vi "pupil find 12 sub vi.vi"(4 "Curve Parameters":T3={"Extraction Mode"=0, "Edge Threshold"=1, "Edge Filter Size"=0, "Min Length"=25, "Row Search Step Size"=10, "Col Search Step Size"=10, "Max Endpoint Gap"=10, "Closed"=FALSE, "Subpixel"=TRUE} {"Max Endpoint Gap" min=0; "Col Search Step Size" min=1 max=255 step=1; "Row Search Step Size" min=1 max=255 step=1; "Min Length" min=0; "Edge Filter Size" items=["Fine", "Normal", "Controur Tracing"]; "Edge Threshold" min=1 max=65535 step=1; "Extraction Mode" items=["Normal", "Uniform Regions"]}, 6 "Circle Descriptor":cluster{"Min Radius":dbl, "Max Radius":dbl}, 7 "New Image 2":T2, 9 "threshold":cluster{"Lower value":sgl, "Upper value":sgl}, 10 "New Image":T2, 11 "Refnum in":T2) -> (0 "Circles":T1(array[cluster]) {"Position"."Y" format="%.2f"; "Position"."X" format="%.2f"}, 1 "Radius":dbl, 2 "Image Dst Out":T2, 3 "Refnum out":T2)   [LabVIEW 2023]
uses:
  <vilib>/vision/Pattern Matching.llb/IMAQ Curve Parameters.ctl
  <vilib>/vision/Image Controls.llb/IMAQ Image.ctl
  <vilib>/vision/Shape Detection.llb/ShapeDetectionMatchOptions.ctl
  <vilib>/vision/Pattern Matching.llb/IMAQ Match Range Setting.ctl
  <vilib>/vision/NI_Vision_Development_Module.lvlib
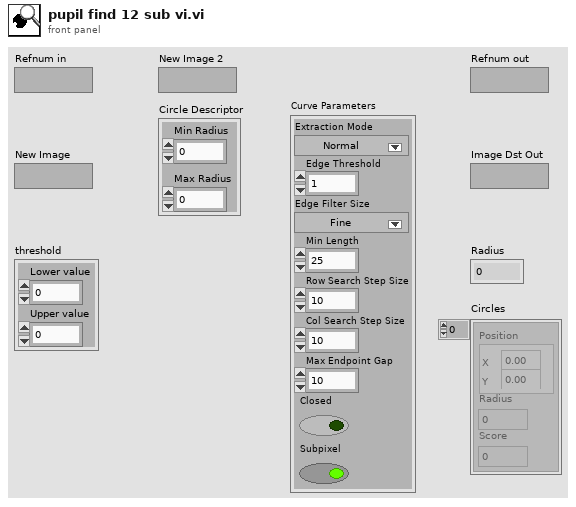
[diagram p1: front panel]
types:
  T1 = cluster{"Position":cluster{"X":sgl, "Y":sgl}, "Radius":dbl, "Score":dbl}[]
  T2 = typedef "IMAQ Image.ctl" = refnum<image>
  T3 = typedef "IMAQ Curve Parameters.ctl" = cluster{"Extraction Mode":u32, "Edge Threshold":i32, "Edge Filter Size":u32, "Min Length":i32, "Row Search Step Size":i32, "Col Search Step Size":i32, "Max Endpoint Gap":i32, "Closed":bool, "Subpixel":bool}
  T4 = typedef "ShapeDetectionMatchOptions.ctl" = cluster{"Rotation":bool, "Scale":bool, "Occlusion":bool, "Range Settings":T5[]}
  T5 = typedef "IMAQ Match Range Setting.ctl" = cluster{"Match Constraints":u32, "Min":dbl, "Max":dbl}
  T6 = typedef "IMAQ Circle" = cluster{"Center X":i32, "Center Y":i32, "Inner Radius":i32, "Outer Radius":i32, "Start Angle":dbl, "End Angle":dbl}
  T7 = typedef "ROI Descriptor" = cluster{"Global Rectangle":i32[], "Contours":cluster{"ID":enum32{"External", "Internal"}, "Type":u32, "Coordinates":i32[]}[]}
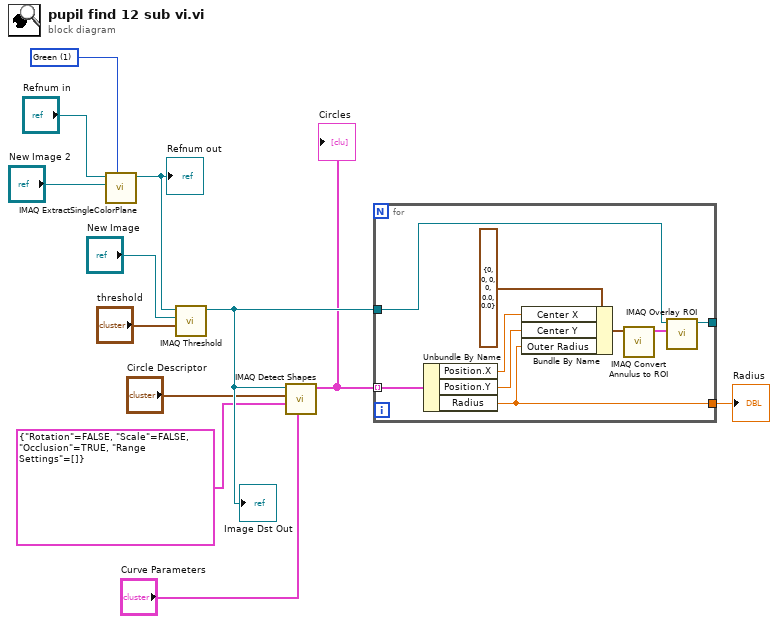
[diagram p0: block diagram]
diagram:
  w1 = 1 items=["Red", "Green", "Blue", "Hue", "Saturation", "Luminance", "Value", "Intensity"] ("Color Plane")
  n1 = call "IMAQ ExtractSingleColorPlane"("Color Plane"=w1, "Image Dst"="New Image 2", "Image Src"="Refnum in") -> ("Image Dst Out"=w6:T2)  [unwired: 7 in, 1 out]
  "Refnum out" <- w6
  n2 = call "IMAQ Threshold"("Range"="threshold", "Image Dst"="New Image", "Image Src"=w6) -> ("Image Dst Out"=w12:T2)  [unwired: 7 in, 1 out]
  "Image Dst Out" <- w12
  n3 = call-poly "IMAQ Detect Shapes"("Curve Parameters"="Curve Parameters", "Match Options"=T4 {"Rotation"=FALSE, "Scale"=FALSE, "Occlusion"=TRUE, "Range Settings"=[]}, "Circle Descriptor"="Circle Descriptor", "Image"=w12) -> ("Circles"=w7:T1)  [unwired: 5 in, 2 out]
  "Circles" <- w7
  n4 = for {
    tunnel: w12 -> [w16]
    tunnel: w7 -> [w15] mode=indexing
    tunnel: [w14] -> _
    tunnel: [w13] -> w11
    n5 = Unbundle By Name(w15) -> ("Position.X"=w19:sgl, "Position.Y"=w18:sgl, "Radius"=w13:dbl)
    n6 = Bundle By Name(cluster=T6 {"Center X"=0, "Center Y"=0, "Inner Radius"=0, "Outer Radius"=0, "Start Angle"=0.0, "End Angle"=0.0} ("Annulus"), "Center X"=w19, "Center Y"=w18, "Outer Radius"=w13) -> (w20:T6)
    n7 = call "IMAQ Convert Annulus to ROI"("Annulus"=w20) -> ("ROI Descriptor"=w17:T7)  [unwired: 8 in, 1 out]
    n8 = call "IMAQ Overlay ROI"("ROI Descriptor"=w17, "Image"=w16) -> ("Image Out"=w14:T2)  [unwired: 8 in, 1 out]
  }
  "Radius" <- w11
